vi "Status Log and Error Handling.vi"(7 "Status Log":refnum<file>, 8 "error in":errorcluster, 10 "Current Bus Number":i32, 11 "Queue in":refnum<queue>) -> (0 "error out":errorcluster, 1 "Current Status":string, 2 "Next State":T1, 3 "Queue out":refnum<queue>, 4 "Status Log":refnum<file>)   [LabVIEW 2014, in "Initialization and IO Node Scripting.lvlib"]
uses:
  Initialization and IO Node Scripting.lvlib
  Scripting States.ctl
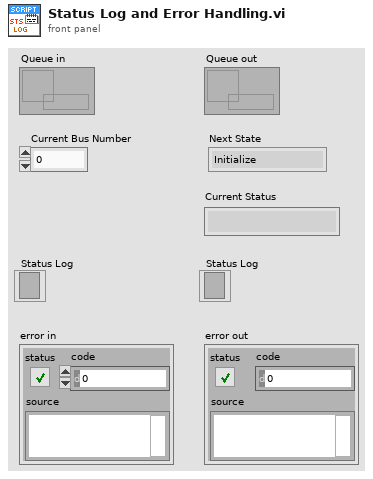
[diagram p1: front panel]
types:
  T1 = typedef "Scripting States.ctl" = enum16{"Initialize", "Modify Dequeue Commands", "Modify Enqueue Data", "Create Project FIFOs", "Create and Place IO Nodes", "Update Node Count in Engine", "Expand FIFO Type Def", "Populate FIFO Names in Engine", "Modify I/O Pin Names", "Modify I/O Pin Enable", "Replace DLU", "Place SPI Engine", "Buses Complete Check", "End"}
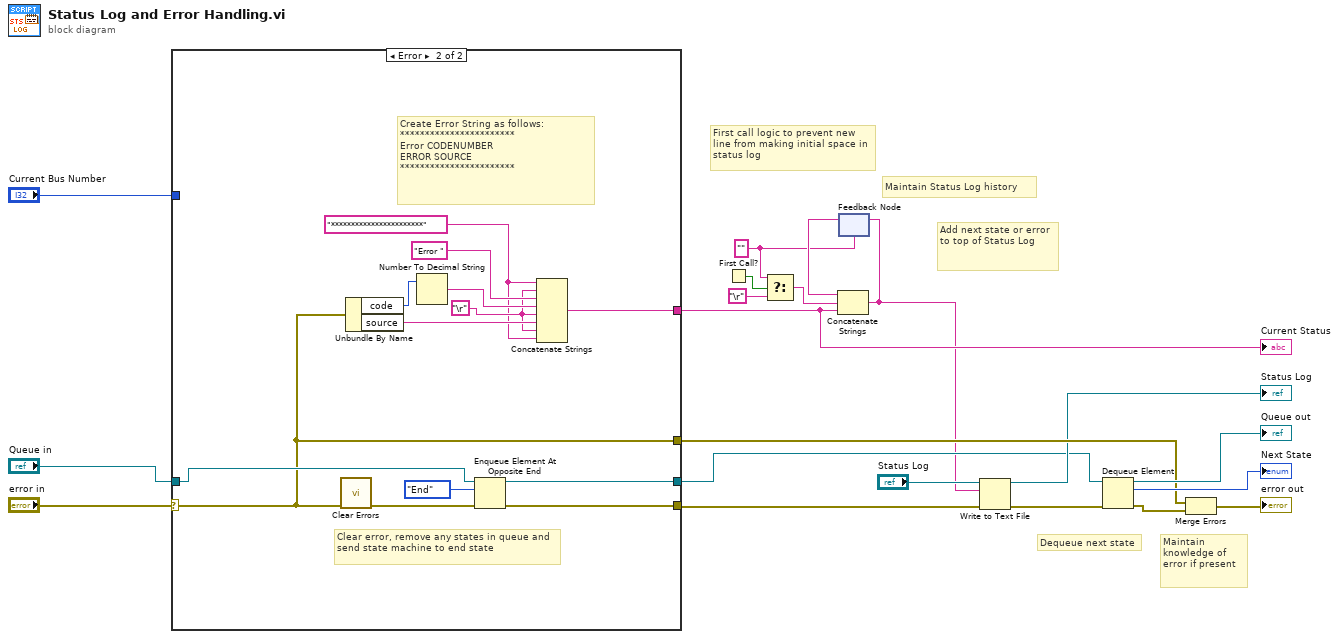
[diagram p0: block diagram]
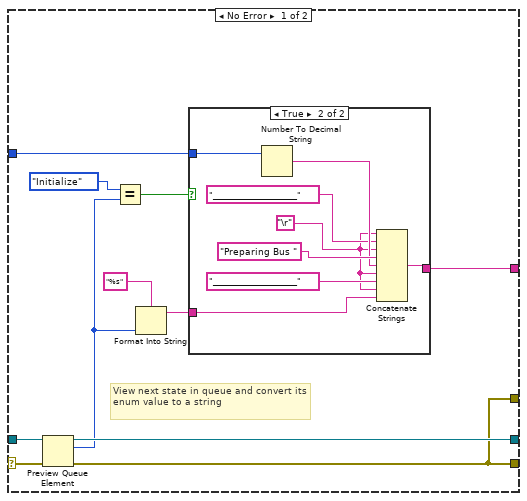
[diagram p2: hidden frame]
diagram:
  w11 = ""
  # "Maintain knowledge of error if present"
  # "Dequeue next state"
  # "Add next state or error to top of Status Log"
  # "Maintain Status Log history"
  # "First call logic to prevent new line from making initial space in status log"
  n1 = case shown="Error" "error in" {
    selector: "error in" -> [w31 w41]
    tunnel: [w23 w50] -> w7
    tunnel: "Queue in" -> [w30 w46]
    tunnel: [w21 w42] -> w6
    tunnel: [w29 w48] -> w2
    tunnel: "Current Bus Number" -> [w25 _]
    tunnel: [w21 w41] -> w8
    frame No Error {
      # "View next state in queue and convert its enum value to a string"
      n2 = Preview Queue Element(queue=w30, error in (no error)=w31) -> (queue out=w29:refnum<queue>, element=w27:T1, error out=w21:errorcluster)  [unwired: 1 in, 1 out]
      n3 = Equal?(x=Scripting_States."Initialize" ("element"), y=w27) -> (x = y?=w24:bool)
      n4 = Format Into String "Format Into String"(format string="%s", w27) -> (resulting string=w22:string)  [unwired: 2 in, 1 out]
      n5 = case shown="True" w24 {
        tunnel: w25 -> [_ w40]
        tunnel: [w32 w39] -> w23
        tunnel: w22 -> [w32 w34]
        frame False {
        }
        frame True {
          w33 = "\r"
          n6 = Number To Decimal String(number=w40) -> (decimal integer string=w37:string)  [unwired: 1 in]
          n7 = Concatenate Strings(w33, "_____________________" ("string"), w33, "Preparing Bus " ("string"), w37, w33, "_____________________" ("string"), w33, w34) -> (w39:string)
        }
      }
    }
    frame Error {
      w43 = "***********************" ("string")
      w44 = "\r"
      # "Create Error String as follows:\n***********************\nError CODENUMBER\nERROR SOURCE\n***********************"
      # "Clear error, remove any states in queue and send state machine to end state"
      n8 = call <vilib>:"Clear Errors.vi"("error in (no error)"=w41) -> ("error out"=w47:errorcluster)  [unwired: 5 in, 1 out]
      n9 = Unbundle By Name(w41) -> ("code"=w51:i32, "source"=w53:string)
      n10 = Number To Decimal String(number=w51) -> (decimal integer string=w52:string)  [unwired: 1 in]
      n11 = Enqueue Element At Opposite End(queue=w46, element=Scripting_States."End", error in (no error)=w47) -> (queue out=w48:refnum<queue>, error out=w42:errorcluster)  [unwired: 1 in, 1 out]
      n12 = Concatenate Strings(w43, w44, "Error " ("string"), w52, w44, w53, w44, w43) -> (w50:string)
    }
  }
  "Current Status" <- w7
  n13 = First Call?() -> (First Call?: T/F=w12:bool)
  n14 = Select(t=w11, s=w12, f="\r") -> (s? t:f=w13:string)
  n15 = feedback #1(w11) -> (w15:string)
  n16 = Concatenate Strings(w15, w13, w7) -> (w1:string)
  n17 = feedback-in #1(w1) -> ()
  n18 = Write to Text File(file (use dialog)="Status Log", text=w1, error in=w6) -> (refnum out=→"Status Log":refnum<file>, error out=w3:errorcluster)  [unwired: 1 in, 1 out]
  n19 = Dequeue Element(queue=w2, error in (no error)=w3) -> (queue out=→"Queue out":refnum<queue>, element=→"Next State":T1, error out=w10:errorcluster)  [unwired: 1 in, 1 out]
  n20 = Merge Errors(w8, w10) -> (→"error out":errorcluster)
